vi "Gear_Gate.vi"(0 "MotorControlDevRef":T1={"DeviceStatus"={"status"=FALSE, "code"=0, "source"=""}, "Type"=enum."PWM", "PWM"={"PWM Channel"=enum."Invalid", "DeadBand"={"Name"="", "maxPositivePwm"=0, "minPositivePwm"=0, "centerPwm"=0, "maxNegativePwm"=0, "minNegativePwm"=0, "angularRange"=0}}, "CAN"={"Device Number"=0, "SetOutput VI Ref"=variant(refnum<vi> refnum), "GetOutput VI Ref"=variant(refnum<vi> refnum), "Enable VI Ref"=variant(refnum<vi> refnum), "Disable VI Ref"=variant(refnum<vi> refnum), "Data"=variant}, "Invert"=FALSE}, 1 "Open_Button_Pressed?":bool, 2 "Close_Button_Pressed?":bool, 3 "Potentiometer_Input":dbl, 4 "Gate_Pos":enum16{"Stop", "Catch", "Clamp", "Open"}(ring), 5 "Acceptable_Range":dbl, 6 "Forward_Limit":dbl, 7 "Forward_StartScale":dbl, 8 "Reverse_Limit":dbl, 9 "Reverse_StartScale":dbl, 10 "Scale_Factor":dbl) -> (14 "Reached":bool)   [LabVIEW 2016]
uses:
  <vilib>/Rock Robotics/WPI/MotorControl/WPI_MotorControlDeviceRef.ctl
  <vilib>/Rock Robotics/WPI/MotorControl/WPI_MotorControlType.ctl
  <vilib>/Rock Robotics/SystemInterfaces/DIO/FPGA_DIOPWMChannel.ctl
  <vilib>/Rock Robotics/WPI/PWM/WPI_PWMDeadband.ctl
panel:
  in  "Open_Pos":dbl
  in  "Clamp_Pos":dbl
  in  "Catch_Pos":dbl
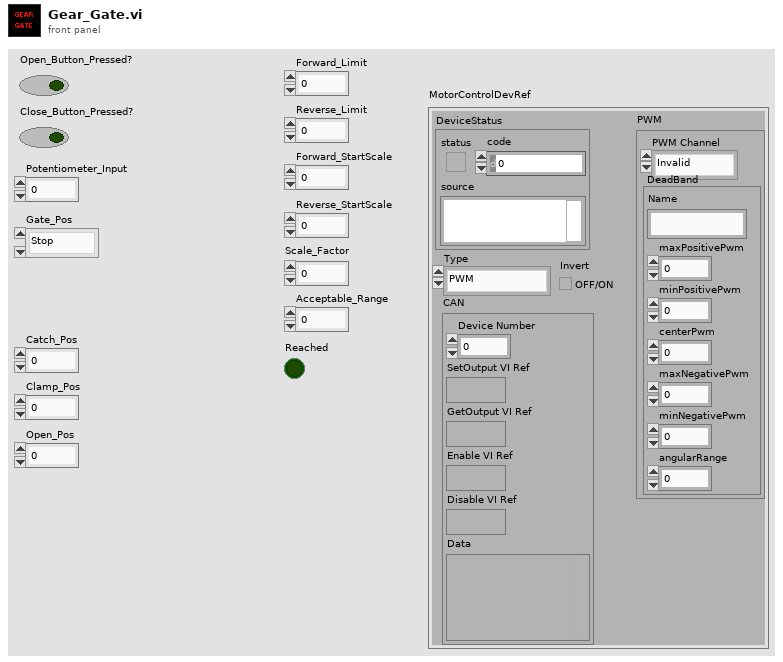
[diagram p1: front panel]
types:
  T1 = typedef "WPI_MotorControlDeviceRef.ctl" = cluster{"DeviceStatus":errorcluster, "Type":T2, "PWM":cluster{"PWM Channel":T3, "DeadBand":T4}, "CAN":cluster{"Device Number":u8, "SetOutput VI Ref":variant, "GetOutput VI Ref":variant, "Enable VI Ref":variant, "Disable VI Ref":variant, "Data":variant}, "Invert":bool}
  T2 = typedef "WPI_MotorControlType.ctl" = enum16{"PWM", "CAN"}
  T3 = typedef "FPGA_DIOPWMChannel.ctl" = enum8{"PWM 0", "PWM 1", "PWM 2", "PWM 3", "PWM 4", "PWM 5", "PWM 6", "PWM 7", "PWM 8", "PWM 9", "PWM MXP 0", "PWM MXP 1", "PWM MXP 2", "PWM MXP 3", "PWM MXP 4", "PWM MXP 5", "PWM MXP 6", "PWM MXP 7", "PWM MXP 8", "PWM MXP 9", "Invalid"}
  T4 = typedef "WPI_PWMDeadband.ctl" = cluster{"Name":string, "maxPositivePwm":i32, "minPositivePwm":i32, "centerPwm":i32, "maxNegativePwm":i32, "minNegativePwm":i32, "angularRange":u16}
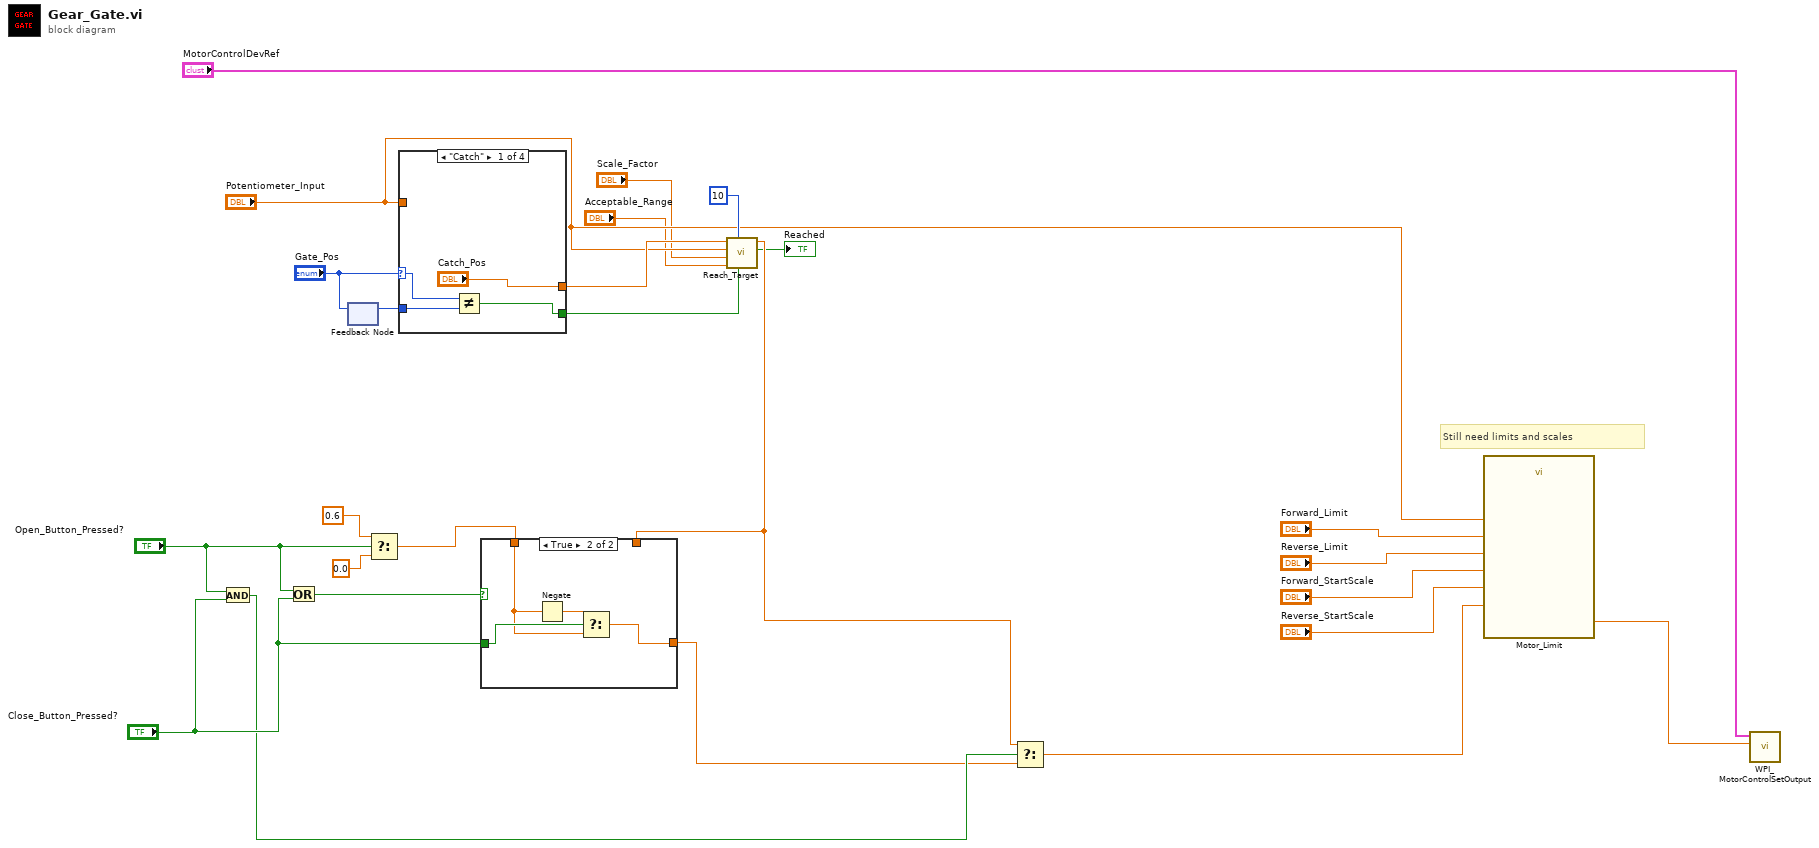
[diagram p0: block diagram]
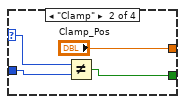
[diagram p3: hidden frame]
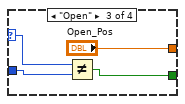
[diagram p4: hidden frame]
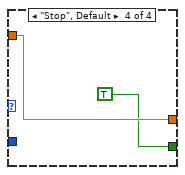
[diagram p5: hidden frame]
diagram:
  # "Still need limits and scales"
  n1 = And(x="Open_Button_Pressed?", y="Close_Button_Pressed?") -> (x .and. y?=w19:bool)
  n2 = Or(x="Open_Button_Pressed?", y="Close_Button_Pressed?") -> (x .or. y?=w20:bool)
  n3 = feedback-in #1("Gate_Pos") -> ()
  n4 = feedback #1() -> (w12:enum16{"Stop", "Catch", "Clamp", "Open"})  [unwired: 1 in]
  n5 = Select(t=0.6, s="Open_Button_Pressed?", f=0.0) -> (s? t:f=w18:dbl)
  n6 = case shown="\"Catch\"" "Gate_Pos" {
    selector: "Gate_Pos" -> [w27 w31 w36 _]
    tunnel: ["Catch_Pos" "Clamp_Pos" "Open_Pos" w39] -> w11
    tunnel: "Potentiometer_Input" -> [_ _ _ w39]
    tunnel: [w28 w32 w34 TRUE] -> w14
    tunnel: w12 -> [w26 w30 w35 _]
    frame "Catch" {
      n7 = Not Equal?(x=w27, y=w26) -> (x != y?=w28:bool)
    }
    frame "Clamp" {
      n8 = Not Equal?(x=w31, y=w30) -> (x != y?=w32:bool)
    }
    frame "Open" {
      n9 = Not Equal?(x=w36, y=w35) -> (x != y?=w34:bool)
    }
    frame "Stop", Default {
    }
  }
  n10 = call "Reach_Target.vi"("Reset"=w14, "Maintain_Samples"=10 ("Num samples"), "Acceptable_Range"="Acceptable_Range", "Scale_Factor"="Scale_Factor", "Current_Position"="Potentiometer_Input", "Target_Position"=w11) -> ("Reached"=→"Reached":bool, "Motor_Value"=w7:dbl)  [unwired: 4 in]
  n11 = case shown="True" w20 {
    tunnel: [w40 w44] -> w17
    tunnel: "Close_Button_Pressed?" -> [_ w43]
    tunnel: w18 -> [_ w41]
    tunnel: w7 -> [w40 _]
    frame False {
    }
    frame True {
      n12 = Negate(x=w41) -> (-x=w42:dbl)
      n13 = Select(t=w42, s=w43, f=w41) -> (s? t:f=w44:dbl)
    }
  }
  n14 = Select(t=w7, s=w19, f=w17) -> (s? t:f=w6:dbl)
  n15 = call "Motor_Limit.vi"("Current_Pos"="Potentiometer_Input", "Motor_Speed"=w6, "Forward_StartScale"="Forward_StartScale", "Reverse_StartScale"="Reverse_StartScale", "Forward_Limit"="Forward_Limit", "Reverse_Limit"="Reverse_Limit") -> ("New_Motor_Speed"=w16:dbl)  [unwired: 13 in]
  n16 = call <vilib>:"WPI_MotorControlSetOutput.vi"("Output"=w16, "MotorControlDevRef"="MotorControlDevRef") -> ()  [unwired: 7 in, 3 out]
